vi "Get measurementservice_ServerEvent.vi"(8 "error in (no error)":errorcluster, 11 "gRPCid":T2) -> (0 "error out":errorcluster, 2 "Message Data":T1, 3 "gRPCid out":T2)   [LabVIEW 2019, in "OCVServer.lvlib" / "OCVServer.lvclass"]
uses:
  OCVServer.lvclass
  gRPC lvSupport/Server API/typeDefs/grpcId.ctl
  measurementservice_ServerEvent_Data.ctl
  a51dd2a7-b5c1-4c09-9df4-8cd9d3bd0c19.vi
  gRPC lvSupport/Server API/Server/Get Server DLL Path.vi
  gRPC lvSupport/gprc-lvsupport.lvlib
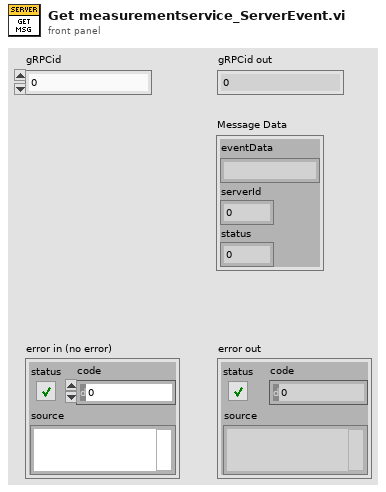
[diagram p1: front panel]
types:
  T1 = typedef "OCVServer.lvlib/OCVServer.lvclass/measurementservice_ServerEvent_Data.ctl" = cluster{"eventData":string, "serverId":i32, "status":i32}
  T2 = typedef "OCVServer.lvlib/gprc-lvsupport.lvlib/grpcId.ctl" = u64
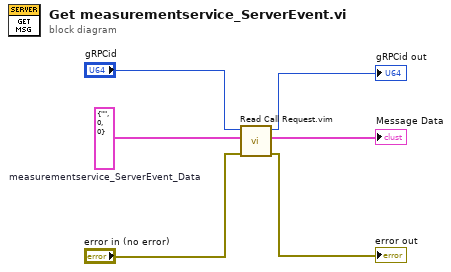
[diagram p0: block diagram]
diagram:
  w2 = T1 {"eventData"="", "serverId"=0, "status"=0}  # measurementservice_ServerEvent_Data
  n1 = call "Read Call Request.vim"("error in (no error)"="error in (no error)", "Data Type"=w2, "gRPCid in"="gRPCid") -> ("error out"=→"error out":errorcluster, "Request Data"=→"Message Data":T1, "gRPCid out"=→"gRPCid out":T2)  [unwired: 6 in]
